vi "Get Instrument List.vi"(8 "error in (no error)":errorcluster, 11 "Instrument Handler in":refnum<class "Instrument Handler.lvclass">) -> (0 "error out":errorcluster, 2 "Instrument Info Array":T1[](array[typedef]), 3 "Instrument Handler out":refnum<class "Instrument Handler.lvclass">)   [LabVIEW 2020, in "Instrument Handler.lvlib" / "Instrument Handler.lvclass"]
doc: "Generate a list of the instruments owned by the Instrument Handler."
uses:
  Instrument Handler.lvclass
  PPL/HDH.Actor Framework.Core.Instrument Driver.lvlibp/Instrument Driver/Controls/Ctl_ConnectionType.ctl
  Controls/Ctl_InstrumentInfo.ctl
  Controls/Ctl_InstrumentSynchronicationCluster.ctl
  PPL/HDH.Data.Generic.lvlibp/Synchronization/Notifier/Notifier.lvclass
  PPL/HDH.Actor Framework.Core.Actor.lvlibp/1abvi3w/vi.lib/ActorFramework/Message Enqueuer/Message Enqueuer.lvclass
  PPL/HDH.Actor Framework.Core.Sequencer.lvlibp/Sequencer Core/Sequencer Core.lvclass
  Instrument Handler.lvclass/Instrument Handler.ctl
  PPL/HDH.Actor Framework.Core.Instrument Driver.lvlibp/Instrument Driver/Instrument Driver.lvclass
  Instrument Handler.lvlib
panel:
  in  "Connection Type":T2=enum."SwitchBlock Device"
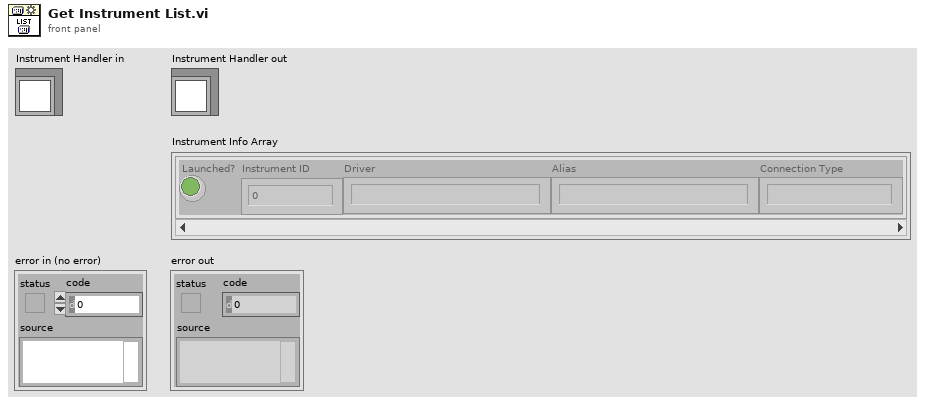
[diagram p1: front panel]
types:
  T1 = typedef "Instrument Handler.lvlib/Ctl_InstrumentInfo.ctl" = cluster{"Launched?":bool, "Instrument ID":u32, "Driver":string, "Alias":string, "Connection Type":string}
  T2 = typedef "HDH.Actor Framework.Core.Instrument Driver.lvlibp/Instrument Driver.lvclass/Ctl_ConnectionType.ctl" = enum16{"BuiltIn/System", "PXI/PCI", "USB", "GPIB", "VXI", "Serial", "TCP/IP", "cRIO", "SCXI", "cDAQ", "SwitchBlock", "SCC", "FireWire", "Accessory", "CAN", "SwitchBlock Device"}
  T3 = typedef "Instrument Handler.lvlib/Ctl_InstrumentSynchronicationCluster.ctl" = cluster{"Launched?":bool, "Driver Path":path, "Alias":string, "Connection Type":T2, "Pre Initialization Data":variant, "Enqueue Sync":refnum<class "Notifier.lvclass">, "Enqueue Lock":T4, "Owner Enqueuer":refnum<class "Message Enqueuer.lvclass">, "Owner":refnum<class "Sequencer Core.lvclass">, "Instrument ID":u32}
  T4 = typedef "Semaphore RefNum" = refnum<k1>
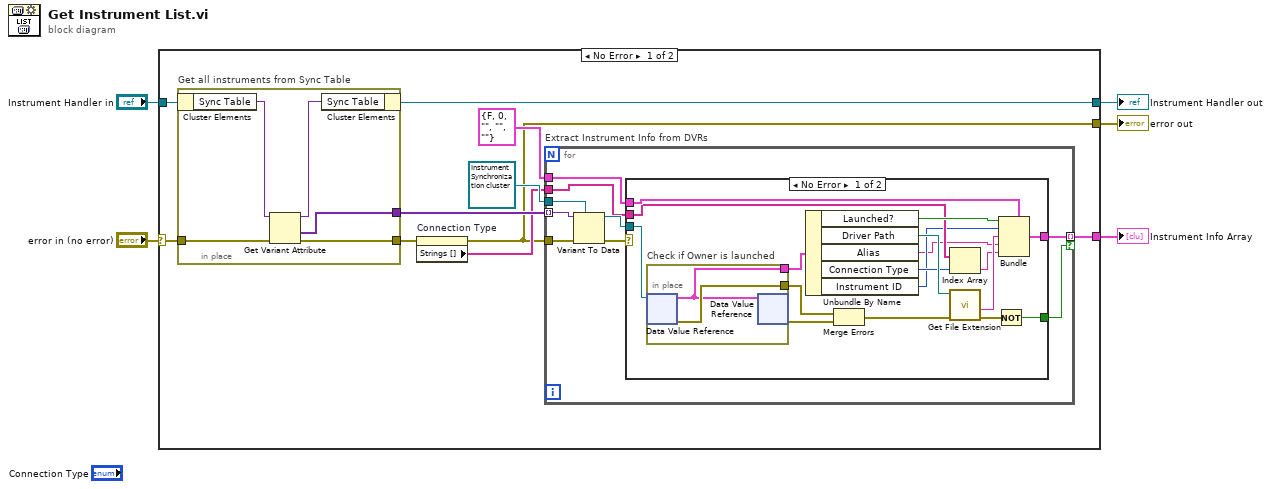
[diagram p0: block diagram]
diagram:
  n1 = case shown="No Error" "error in (no error)" {
    selector: "error in (no error)" -> [w13 w50]
    tunnel: [w6 w50] -> w4
    tunnel: [w14 w49] -> w2
    tunnel: "Instrument Handler in" -> [w15 w49]
    tunnel: [w7 _] -> w1
    frame No Error {
      n2 = in-place "Get all instruments from Sync Table" {
        in-place-border: w13 -> [w46]
        in-place-border: [w45] -> w10
        in-place-border: [w44] -> w12
        n3 = in-place-cluster #1(w15) -> ("Sync Table"=w48:variant)
        n4 = Get Variant Attribute(Variant=w48, error in=w46) -> (duplicate Variant=w47:variant, values=w44:variant[], error out=w45:errorcluster)  [unwired: 2 in, 1 out]
        n5 = in-place-cluster #1("Sync Table"=w47) -> (w14:refnum<class "Instrument Handler.lvclass">)
      }
      n6 = property on="Connection Type" class="Enum (strict)"(error in=w10) -> (error out=w6:errorcluster, "Strings []"=w9:string[])  [unwired: 1 in, 1 out]
      n7 = for "Extract Instrument Info from DVRs" {
        tunnel: w12 -> [w24] mode=indexing
        tunnel: refnum<data-value> refnum ("data value reference") -> [w23]
        tunnel: w9 -> [w20]
        tunnel: T1 {"Launched?"=FALSE, "Instrument ID"=0, "Driver"="", "Alias"="", "Connection Type"=""} ("Instrument Info") -> [w19]
        tunnel: [w18] -> w7 mode=indexing if=w17
        tunnel: w6 -> [w16]
        n8 = Variant To Data(error in=w16, type=w23, Variant=w24) -> (data=w21:refnum<data-value>, error out=w22:errorcluster)
        n9 = case shown="No Error" w22 {
          tunnel: w21 -> [w41 _]
          tunnel: w20 -> [w34 _]
          tunnel: w19 -> [w38 _]
          tunnel: [w31 _] -> w18
          tunnel: [w29 _] -> w17
          frame No Error {
            n10 = in-place "Check if Owner is launched" {
              in-place-border: [w43] -> w39
              in-place-border: [w42] -> w37
              n11 = in-place-dvr #2(w41) -> (w42:T3, w43:errorcluster)
              n12 = in-place-dvr #2(w42) -> (w40:errorcluster)  [unwired: 1 out]
            }
            n13 = Unbundle By Name(w37) -> ("Launched?"=w36:bool, "Driver Path"=w35:path, "Alias"=w26:string, "Connection Type"=w32:T2, "Instrument ID"=w28:u32)
            n14 = Merge Errors(w39, w40) -> (w33:errorcluster)
            n15 = Index Array(array=w34, index=w32) -> (element=w25:string)
            n16 = call <vilib>:"Get File Extension.vi"("error in (no error)"=w33, "file"=w35) -> ("error out"=w30:errorcluster, "filename without extension"=w27:string)  [unwired: 5 in, 3 out]
            n17 = Not(x=w30) -> (.not. x?=w29:bool)
            n18 = Bundle(cluster=w38, "Launched?"=w36, "Instrument ID"=w28, "Driver"=w27, "Alias"=w26, "Connection Type"=w25) -> (w31:T1)
          }
          frame Error {
          }
        }
      }
    }
    frame Error {
    }
  }
  "error out" <- w4
  "Instrument Handler out" <- w2
  "Instrument Info Array" <- w1
